vi "Modbus Multi-Read U16.vi"(7 "Slave Address":u8, 8 "error in (no error)":errorcluster, 9 "Number of U16 to read":i32 format="%x", 10 "Register Start Address":u16 format="%x", 11 "VISA resource in":refnum<visa-resource-name>) -> (0 "error out":errorcluster, 1 "Output data [U16]":u16[](array[numeric]), 3 "VISA resource out":refnum<visa-resource-name>)   [LabVIEW 2023, in "Voegtlin_NI_SMART_Modbus_Drivers.lvlib"]
doc: "Lese die geforderte Anzahl U16-Werte ab der angegebenen Startadresse des selektierten Geraetes aus.\nDer COM-Port muss dazu initialisiert sein (benutze\" Modbus Init.vi\")."
uses:
  Voegtlin_NI_SMART_Modbus_Drivers.lvlib
  Enums/Modbus Comm.ctl
panel:
  out "Read register data\n U16 (array)":u16[](array[numeric])
  # "Internal Data"
  # "Output Data"
  # "Input Data"
  # "(Inputmaske in HEX)"
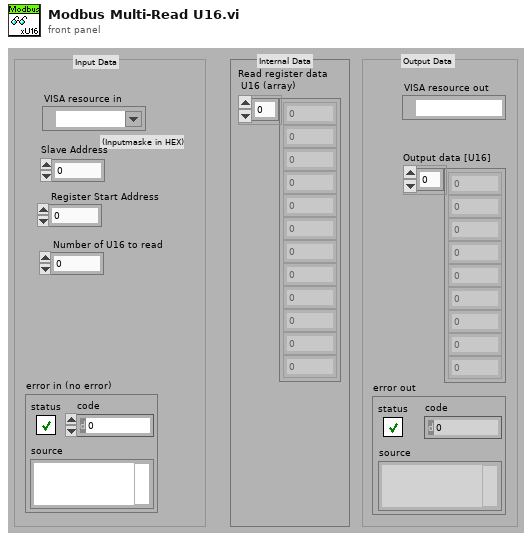
[diagram p1: front panel]
types:
  T1 = typedef "Voegtlin_NI_SMART_Modbus_Drivers.lvlib/Modbus Comm.ctl" = enum16{"Init", "Read", "Write", "Exit"}
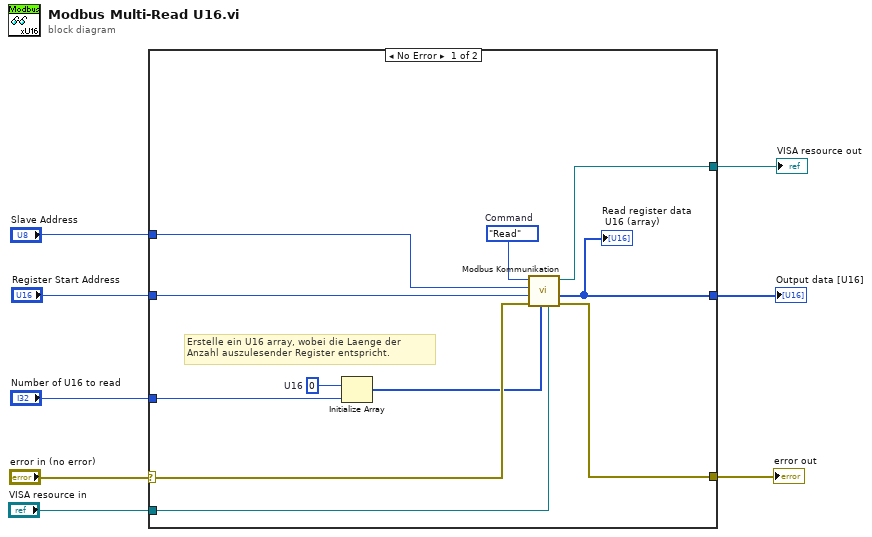
[diagram p0: block diagram]
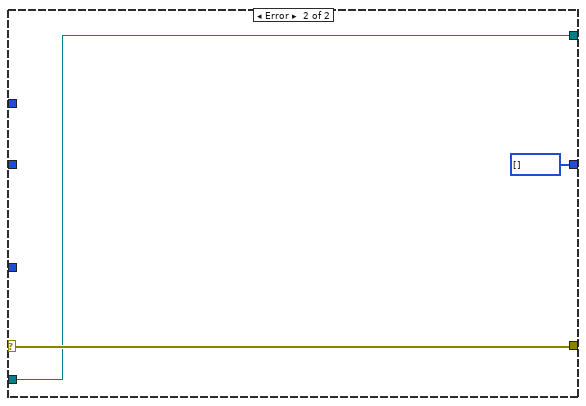
[diagram p2: hidden frame]
diagram:
  n1 = case shown="No Error" "error in (no error)" {
    selector: "error in (no error)" -> [w14 w22]
    tunnel: "Register Start Address" -> [w12 _]
    tunnel: [w19 w22] -> w7
    tunnel: "Number of U16 to read" -> [w16 _]
    tunnel: [w15 u16[] [] ("Data Out (array)")] -> w5
    tunnel: "Slave Address" -> [w11 _]
    tunnel: "VISA resource in" -> [w10 w20]
    tunnel: [w9 w20] -> w1
    frame No Error {
      w17 = u16 0  # U16
      w18 = Modbus_Comm."Read"  # Command
      # "Erstelle ein U16 array, wobei die Laenge der Anzahl auszulesender Register entspricht."
      n2 = Initialize Array(w17, w16) -> (w13:u16[])
      n3 = call "Modbus Kommunikation.vi"("VISA resource in"=w10, "Data In / #Reads [U16]"=w13, "error in (no error)"=w14, "Register Start Address"=w12, "Slave Address"=w11, "Command"=w18) -> ("error out"=w19:errorcluster, "Data Out [U16]"=w15:u16[], "VISA resource out"=w9:refnum<visa-resource-name>)  [unwired: 3 in]
      "Read register data\n U16 (array)" <- w15
    }
    frame Error {
    }
  }
  "error out" <- w7
  "Output data [U16]" <- w5
  "VISA resource out" <- w1
